vi "Square_Pulse(SubVI).vi"(6 "High Voltage (V)":dbl, 9 "Pulse Width":dbl, 10 "Pulse Start (us)":dbl, 11 "Time":dbl) -> (2 "Voltage Out":dbl, 3 "unsigned 16-bit out":u16)   [LabVIEW 2016]
panel:
  in  "Pulse Width":dbl format="%#_13g"
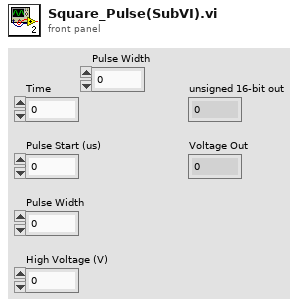
[diagram p1: front panel]
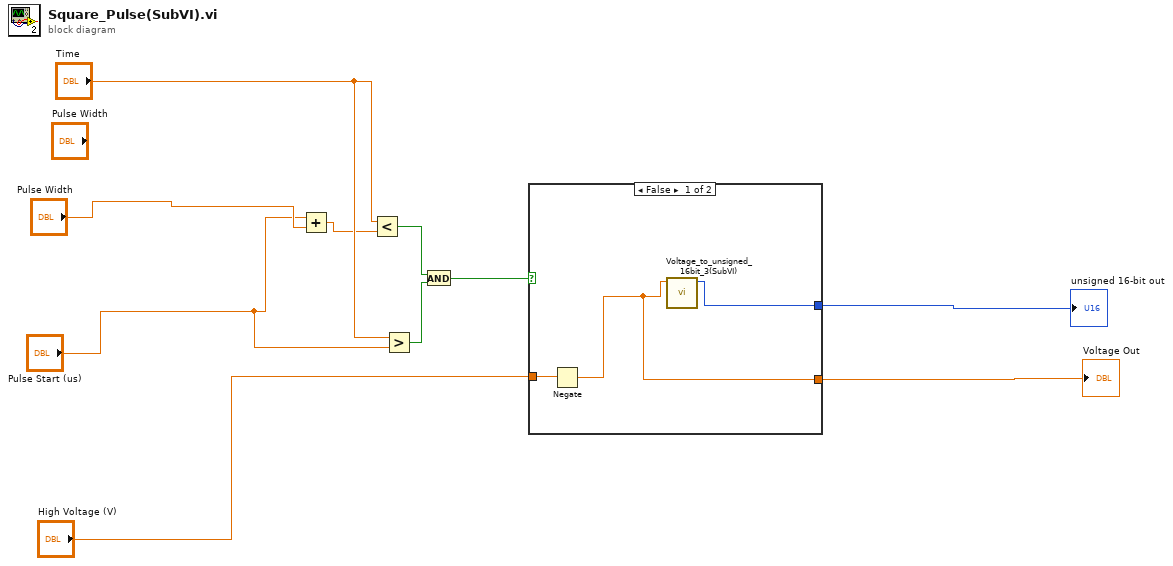
[diagram p0: block diagram]
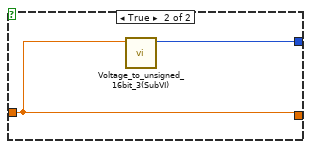
[diagram p2: hidden frame]
diagram:
  n1 = Add(x="Pulse Start (us)", y="Pulse Width") -> (x+y=w3:dbl)
  n2 = Less?(x="Time", y=w3) -> (x < y?=w5:bool)
  n3 = Greater?(x="Time", y="Pulse Start (us)") -> (0:w6:bool)
  n4 = And(x=w5, y=w6) -> (x .and. y?=w7:bool)
  n5 = case shown="False" w7 {
    tunnel: "High Voltage (V)" -> [w12 w14]
    tunnel: [w13 w15] -> w9
    tunnel: [w11 w14] -> w10
    frame False {
      n6 = Negate(x=w12) -> (-x=w11:dbl)
      n7 = call "Voltage_to_unsigned_16bit_3(SubVI).vi"("Voltage_in"=w11) -> ("unsigned 16bit integer"=w13:u16)  [unwired: 10 in]
    }
    frame True {
      n8 = call "Voltage_to_unsigned_16bit_3(SubVI).vi"("Voltage_in"=w14) -> ("unsigned 16bit integer"=w15:u16)  [unwired: 10 in]
    }
  }
  "unsigned 16-bit out" <- w9
  "Voltage Out" <- w10
